vi "Temperature Monitor.vi"(7 "Temperature Threshhold":dbl, 9 "Notification":string, 10 "DMM In":string, 11 "Sequence Context In":refnum<k7>) -> (0 "error out":errorcluster, 2 "Temperature Data":dbl[][](array[numeric]), 3 "Thermal Event":bool)   [LabVIEW 2013]
uses:
  <instrlib>/Driver Simulation/DMM/TemperatureSensorTypes.ctl
  <vilib>/addons/TestStand/_TSUtility.llb/TestStand - Get Property Value (Number {Signed 32-bit Integer}).vi
  <vilib>/addons/TestStand/_TSUtility.llb/TestStand - Get Property Value (String).vi
  <instrlib>/Driver Simulation/DMM.lvlib
panel:
  out "UUT Serial:":string
  out "Current UUT Temperature":T1(graph)
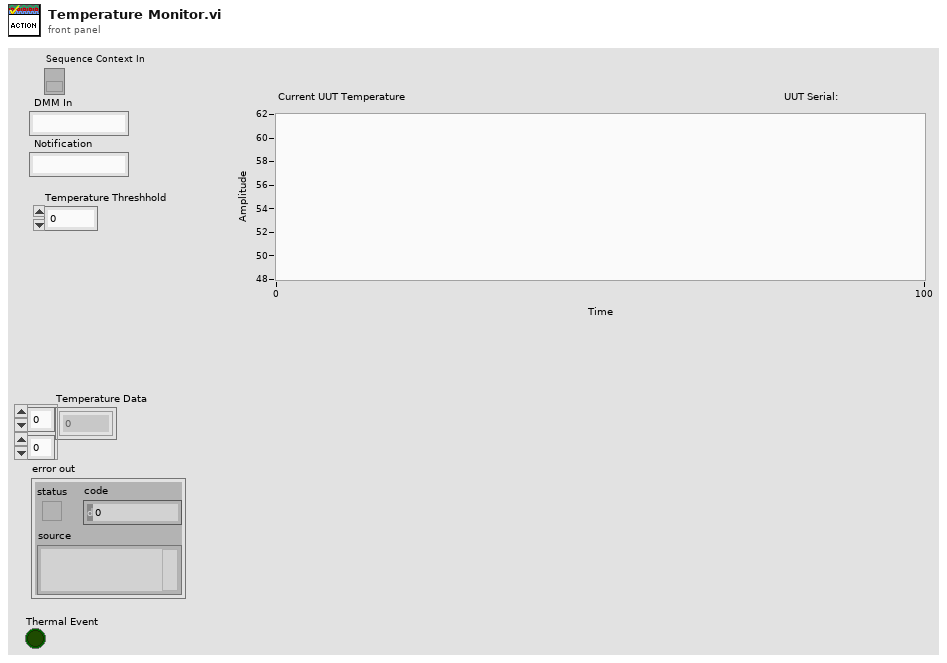
[diagram p1: front panel]
types:
  T1 = cluster{"Temperature (C)":dbl, "Temperature Threshhold":dbl}
  T2 = cluster{"Temperature (C)":dbl, "Temperature Threshhold":dbl}[]
  T3 = typedef "TestStand - Status Monitor.ctl" = cluster{"Sequence Context":refnum<k7>, "Execution":refnum<k7>, "Termination Monitor":refnum<k7>}
  T4 = typedef "Driver Simulation.lvlib/DMM.lvlib/TemperatureSensorTypes.ctl" = i32
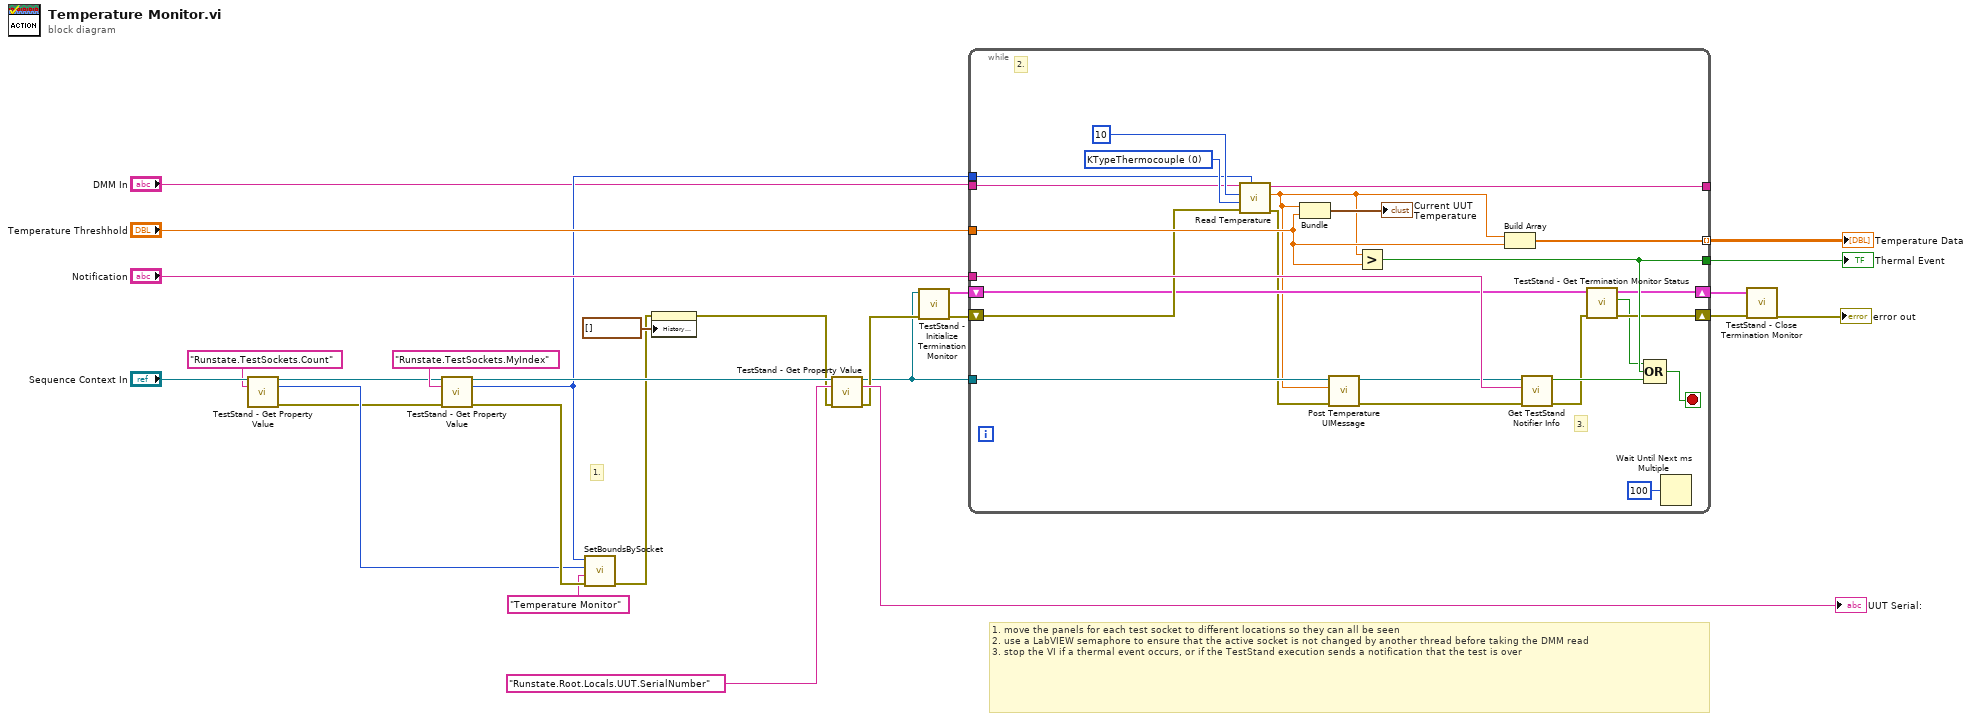
[diagram p0: block diagram]
diagram:
  # "1. move the panels for each test socket to different locations so they can all be seen\n2. use a LabVIEW semaphore to ensure that the active socket is not changed by another thread before taking the DMM read\n3. stop the VI if a thermal event occurs, or if the TestStand execution sends a notification that the test is over"
  # "1."
  n1 = call-poly <vilib>:"TestStand - Get Property Value.vi"("Sequence Context In"="Sequence Context In", "Lookup String"="Runstate.TestSockets.Count") -> ("Sequence Context Out"=w14:refnum<k7>, "Value"=w11:i32, "error out"=w10:errorcluster)  [unwired: 11 in]
  n2 = call-poly <vilib>:"TestStand - Get Property Value.vi"("Sequence Context In"=w14, "Lookup String"="Runstate.TestSockets.MyIndex", "error in (no error)"=w10) -> ("Sequence Context Out"=w20:refnum<k7>, "Value"=w16:i32, "error out"=w18:errorcluster)  [unwired: 10 in]
  n3 = call "SetBoundsBySocket.vi"("Error In"=w18, "Test Name"="Temperature Monitor", "Number of Sockets"=w11, "Test Socket"=w16) -> ("Error Out"=w17:errorcluster)  [unwired: 7 in]
  n4 = property on="Current UUT Temperature" class="WFChart (strict)"(error in=w17, "History Data"=T2 []) -> (error out=w8:errorcluster)  [unwired: 1 in, 1 out]
  n5 = call-poly <vilib>:"TestStand - Get Property Value.vi"("Sequence Context In"=w20, "Lookup String"="Runstate.Root.Locals.UUT.SerialNumber", "error in (no error)"=w8) -> ("Sequence Context Out"=w1:refnum<k7>, "Value"=→"UUT Serial:":string, "error out"=w6:errorcluster)  [unwired: 10 in]
  n6 = call <vilib>:"TestStand - Initialize Termination Monitor.vi"("error in (no error)"=w6, "Sequence Context In"=w1) -> ("error out"=w7:errorcluster, "Status Monitor Out"=w5:T3)  [unwired: 8 in]
  n7 = while {
    tunnel: w1 -> [w32]
    tunnel: "DMM In" -> [w38]
    tunnel: "Notification" -> [w51]
    shift-right: [w36] -> w4
    shift-left: w7 -> [w39]
    tunnel: "Temperature Threshhold" -> [w45]
    tunnel: [w48] -> w25
    tunnel: [w43] -> w24 mode=indexing
    tunnel: w16 -> [w40]
    tunnel: [w41] -> _
    shift-right: [w34] -> w2
    shift-left: w5 -> [w33]
    stop <- w46 stop-if-true
    w50 = T4 0 items=["KTypeThermocouple", "JTypeThermocouple"] ("sensorType")
    # "2."
    # "3."
    n8 = call <instrlib>:"Read Temperature.vi"("Test Socket (0)"=w40, "error in (no error)"=w39, "Sensor Type"=w50, "Channel"=10 ("DMM Channel"), "DMM in"=w38) -> ("error out"=w30:errorcluster, "Temperature (C)"=w31:dbl, "DMM out"=w41:string)  [unwired: 4 in]
    n9 = Bundle("Temperature (C)"=w31, "Temperature Threshhold"=w45) -> (→"Current UUT Temperature":T1)  [unwired: 1 in]
    n10 = call "Post Temperature UIMessage.vi"("error in (no error)"=w30, "Temperature"=w31, "SequenceContext in"=w32) -> ("error out"=w29:errorcluster, "SequenceContext out"=w28:refnum<k7>)  [unwired: 7 in]
    n11 = Greater?(x=w31, y=w45) -> (0:w48:bool)
    n12 = Build Array(w31, w45) -> (w43:dbl[])
    n13 = call "Get TestStand Notifier Info.vi"("error in (no error)"=w29, "Notifier"=w51, "SequenceContext"=w28) -> ("error out"=w37:errorcluster, "Stop"=w47:bool)  [unwired: 7 in]
    n14 = call <vilib>:"TestStand - Get Termination Monitor Status.vi"("error in (no error)"=w37, "Status Monitor In"=w33) -> ("error out"=w36:errorcluster, "Terminating or Aborting"=w35:bool, "Status Monitor Out"=w34:T3)  [unwired: 7 in]
    n15 = Compound Arithmetic op=OR(w35, w48, w47) -> (w46:bool)
    n16 = Wait Until Next ms Multiple(millisecond multiple=u32 100) -> ()  [unwired: 1 out]
  }
  "Thermal Event" <- w25
  "Temperature Data" <- w24
  n17 = call <vilib>:"TestStand - Close Termination Monitor.vi"("error in (no error)"=w4, "Status Monitor In"=w2) -> ("error out"=→"error out":errorcluster)  [unwired: 9 in]
